vi "FGV_DrapAndDrop_Data.vi"(7 "Modes":T1, 8 "error in (no error)":errorcluster, 9 "Target String Element Ref":refnum<vi>, 10 "Channel Name":string) -> (0 "error out":errorcluster, 1 "Target String Element Ref Out":refnum<vi>, 2 "Channel Name Out":string)   [LabVIEW 2018]
uses:
  TypeDefs/TD_Case_SimpleFGVModes.ctl
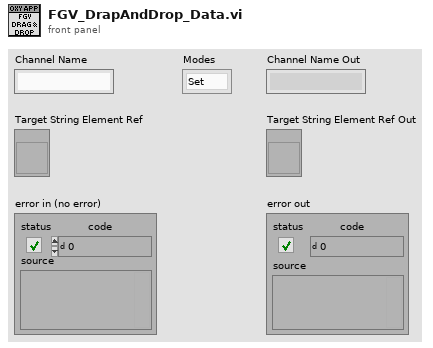
[diagram p1: front panel]
types:
  T1 = typedef "TD_Case_SimpleFGVModes.ctl" = enum16{"Set", "Get"}
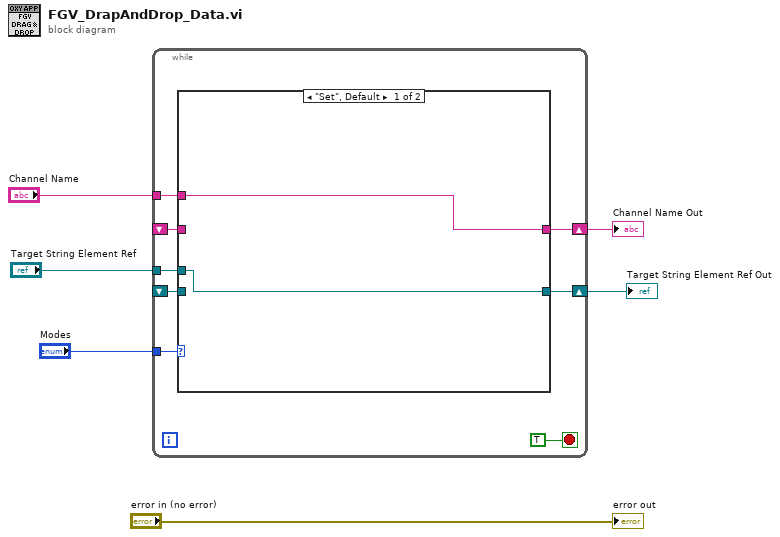
[diagram p0: block diagram]
diagram:
  n1 = while {
    tunnel: "Modes" -> [w14]
    tunnel: "Channel Name" -> [w12]
    shift-right: [w11] -> w2
    shift-left: _ -> [w8]
    tunnel: "Target String Element Ref" -> [w10]
    shift-right: [w9] -> w1
    shift-left: _ -> [w7]
    stop <- TRUE stop-if-true
    n2 = case shown="\"Set\", Default" w14 {
      tunnel: w12 -> [w16 _]
      tunnel: [w16 w18] -> w11
      tunnel: w10 -> [w15 _]
      tunnel: [w15 w17] -> w9
      tunnel: w8 -> [_ w18]
      tunnel: w7 -> [_ w17]
      frame "Set", Default {
      }
      frame "Get" {
      }
    }
  }
  "Target String Element Ref Out" <- w1
  "Channel Name Out" <- w2
  "error out" <- "error in (no error)"
